vi "Configure Tag Voltage Pulse (Linear).vi"(0 "VISA resource name":refnum<visa-resource-name>, 1 "Source Measure Unit Channel (0:  Channel A)":i32(ring) items=[" Channel A", " Channel B"], 2 "Bias Level (0 A)":dbl, 3 "Current Limit (1 A)":dbl=1.0, 4 "Current Buffer (smua.nvbuffer1)":string="smua.nvbuffer1", 5 "Pulse Start Level (1 V)":dbl=1.0, 6 "Pulse Stop Level (10 V)":dbl=10.0, 7 "error in (no error)":errorcluster, 8 "Pulse Train Tag (1)":i32=1, 9 "Pulse On Time (0.02 S)":dbl=0.02, 10 "Pulse Measure Cycles (10)":i32=10, 11 "Pulse Off Time (0.04 S)":dbl=0.04, 12 "Trigger Input (0)":i32, 13 "Trigger Wait Time (10 S)":dbl=10.0, 14 "Trigger Output (0)":i32, 15 "Missing Trigger (0: Nil)":i32(ring) items=["Nil", "Abort Pulse", "Not Abort Pulse"]) -> (20 "VISA resource name out":refnum<visa-resource-name>, 27 "error out":errorcluster)   [LabVIEW 2015, in "Keithley 2600 Series.lvlib"]
doc: "Configures a linear pulsed voltage sweep with a current measurement.\n\n<b>Note:</b>\nThis VI does not cause the specified source measure unit channel to output a pulse train. It simply checks to see if all the pulse dimensions can be achieved, and if they are, assigns the indicated pulse train tag to the pulse train. You need to call <b>Initiate Pulse Test</b> VI to initiate a pulse train."
uses:
  Keithley 2600 Series.lvlib
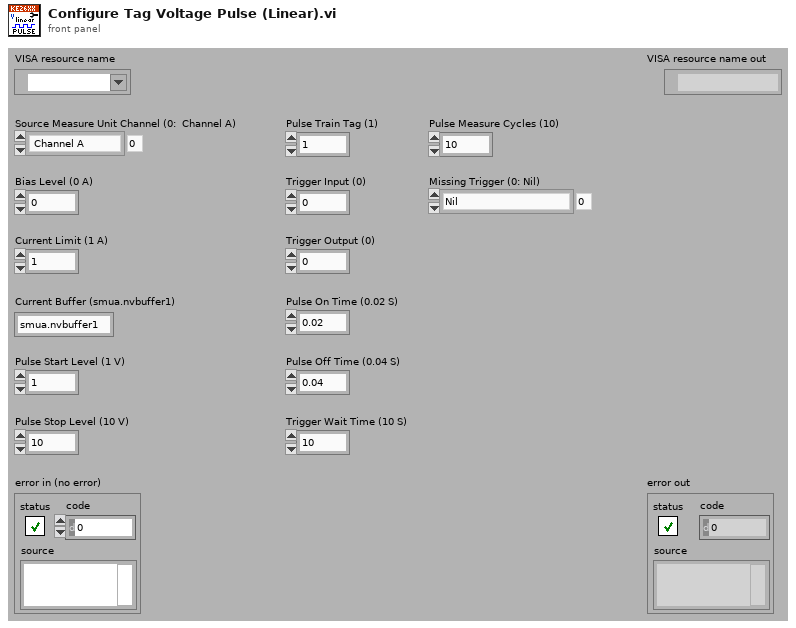
[diagram p1: front panel]
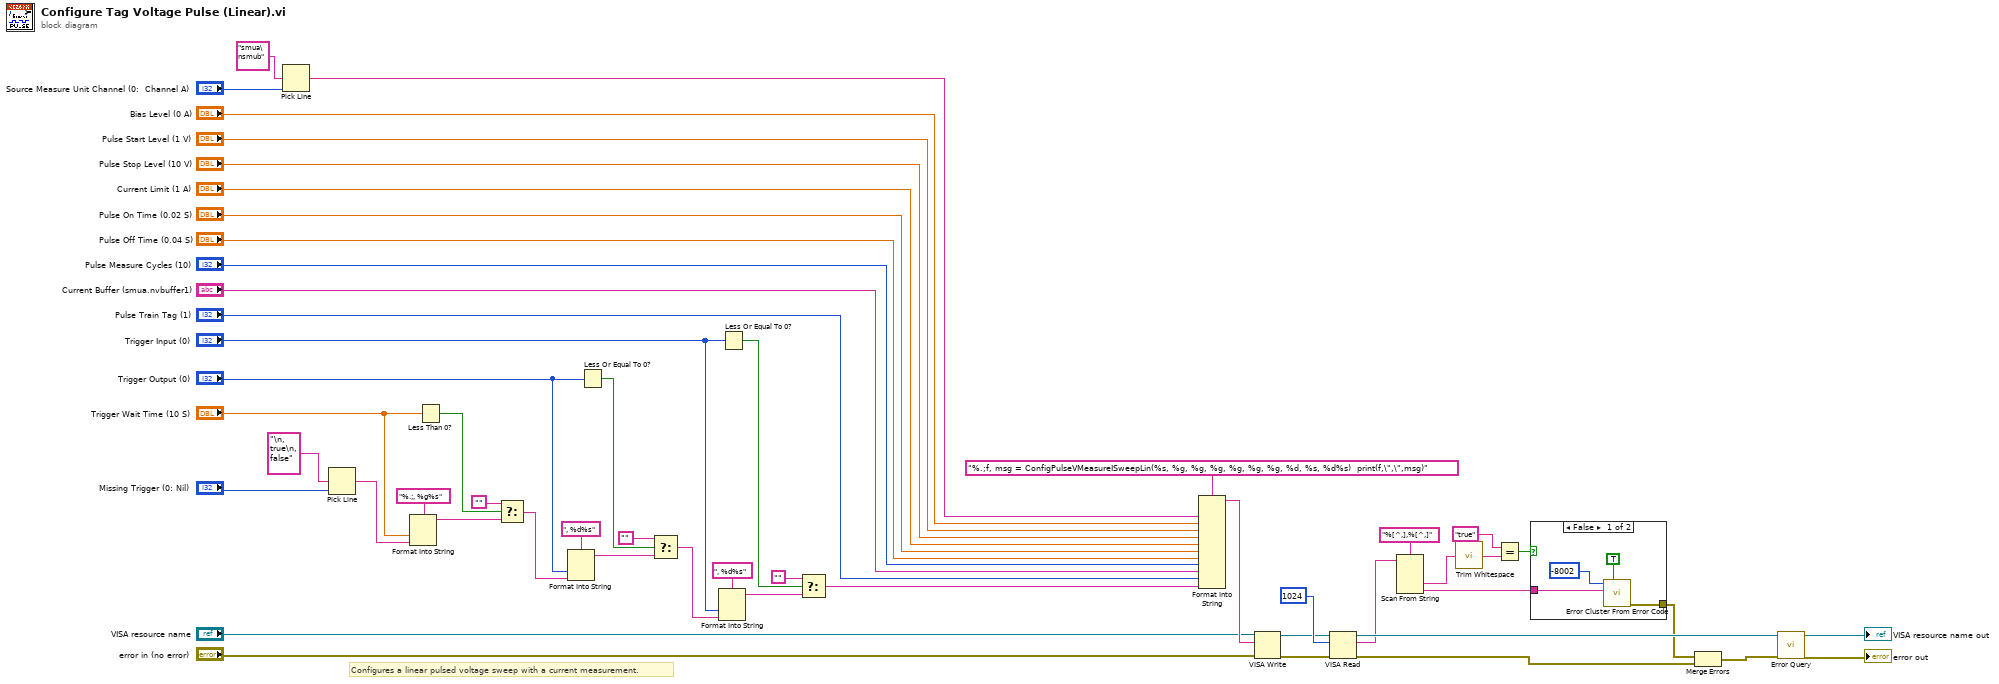
[diagram p0: block diagram]
diagram:
  # "Configures a linear pulsed voltage sweep with a current measurement."
  n1 = Pick Line(multi-line string="smua\nsmub", line index="Source Measure Unit Channel (0:  Channel A)") -> (output string=w46:string)  [unwired: 1 in]
  n2 = Pick Line(multi-line string="\n, true\n, false", line index="Missing Trigger (0: Nil)") -> (output string=w10:string)  [unwired: 1 in]
  n3 = Format Into String(format string="%.;, %g%s", "Trigger Wait Time (10 S)", w10) -> (resulting string=w14:string)  [unwired: 2 in, 1 out]
  n4 = Less Than 0?(x="Trigger Wait Time (10 S)") -> (x < 0?=w20:bool)
  n5 = Select(t="", s=w20, f=w14) -> (s? t:f=w11:string)
  n6 = Format Into String(format string=", %d%s", "Trigger Output (0)", w11) -> (resulting string=w16:string)  [unwired: 2 in, 1 out]
  n7 = Less Or Equal To 0?(x="Trigger Output (0)") -> (x <= 0?=w22:bool)
  n8 = Select(t="", s=w22, f=w16) -> (s? t:f=w12:string)
  n9 = Format Into String(format string=", %d%s", "Trigger Input (0)", w12) -> (resulting string=w13:string)  [unwired: 2 in, 1 out]
  n10 = Less Or Equal To 0?(x="Trigger Input (0)") -> (x <= 0?=w25:bool)
  n11 = Select(t="", s=w25, f=w13) -> (s? t:f=w5:string)
  n12 = Format Into String(format string="%.;f, msg = ConfigPulseVMeasureISweepLin(%s, %g, %g, %g, %g, %g, %g, %d, %s, %d%s)  print(f,\",\",msg)", w46, "Bias Level (0 A)", "Pulse Start Level (1 V)", "Pulse Stop Level (10 V)", "Current Limit (1 A)", "Pulse On Time (0.02 S)", "Pulse Off Time (0.04 S)", "Pulse Measure Cycles (10)", "Current Buffer (smua.nvbuffer1)", "Pulse Train Tag (1)", w5) -> (resulting string=w52:string)  [unwired: 2 in, 1 out]
  n13 = VISA Write(VISA resource name="VISA resource name", write buffer=w52, error in (no error)="error in (no error)") -> (VISA resource name out=w36:refnum<visa-resource-name>, error out=w35:errorcluster)  [unwired: 1 out]
  n14 = VISA Read(VISA resource name=w36, byte count=u32 1024, error in (no error)=w35) -> (VISA resource name out=w34:refnum<visa-resource-name>, read buffer=w26:string, error out=w3:errorcluster)  [unwired: 1 out]
  n15 = Scan From String(format string="%[^,],%[^,]", input string=w26) -> (output 1=w31:string, output 2=w27:string)  [unwired: 4 in, 3 out]
  n16 = call <vilib>:"Trim Whitespace.vi"("string"=w31) -> ("trimmed string"=w30:string)  [unwired: 1 in]
  n17 = Equal?(x="true", y=w30) -> (x = y?=w28:bool)
  n18 = case shown="False" w28 {
    tunnel: [w55 _] -> w4
    tunnel: w27 -> [w57 _]
    frame False {
      n19 = call <vilib>:"Error Cluster From Error Code.vi"("show call chain? (False)"=TRUE, "error message (\"\")"=w57, "error code (0)"=-8002) -> ("error out"=w55:errorcluster)  [unwired: 6 in]
    }
    frame True {
    }
  }
  n20 = Merge Errors(w4, w3) -> (w2:errorcluster)
  n21 = call "Error Query.vi"("error in (no error)"=w2, "VISA resource name"=w34) -> ("error out"=→"error out":errorcluster, "VISA resource name out"=→"VISA resource name out":refnum<visa-resource-name>)  [unwired: 6 in, 2 out]
